vi "Thermocouple.vi"(3 "cj(mV)":dbl, 4 "factor":dbl, 5 "data":dbl) -> (0 "hot(mV)":dbl, 1 "tc(mV)":dbl, 2 "temp(degC)":dbl)   [LabVIEW 2014]
panel:
  in  "offset":dbl
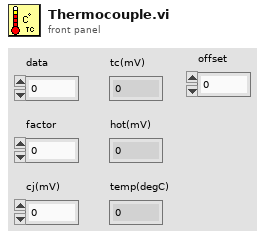
[diagram p1: front panel]
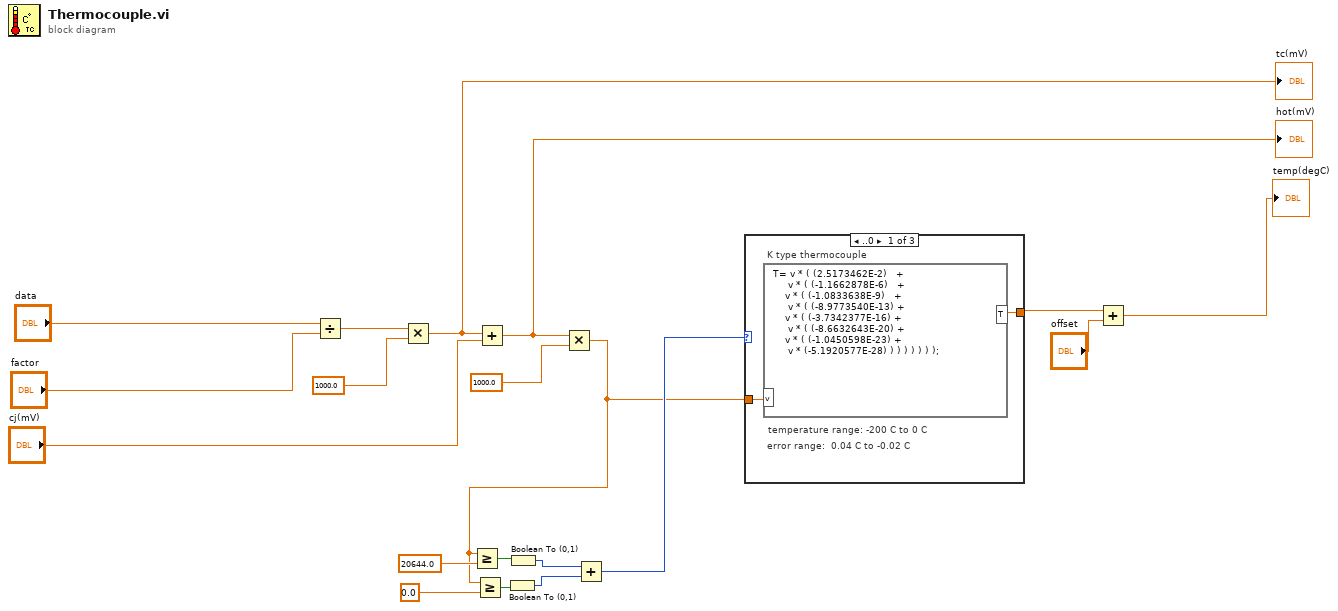
[diagram p0: block diagram]
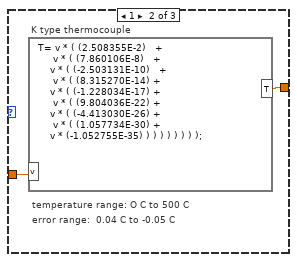
[diagram p2: hidden frame]
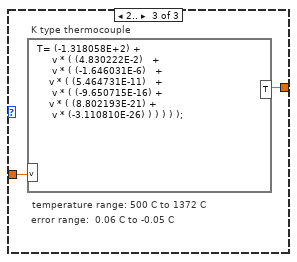
[diagram p3: hidden frame]
diagram:
  n1 = Divide(x="data", y="factor") -> (x/y=w6:dbl)
  n2 = Multiply(x=w6, y=1000.0) -> (x*y=w4:dbl)
  "tc(mV)" <- w4
  n3 = Add(x=w4, y="cj(mV)") -> (x+y=w7:dbl)
  "hot(mV)" <- w7
  n4 = Multiply(x=w7, y=1000.0) -> (x*y=w8:dbl)
  n5 = Greater Or Equal?(x=w8, y=20644.0) -> (x >= y?=w14:bool)
  n6 = Greater Or Equal?(x=w8, y=0.0) -> (x >= y?=w13:bool)
  n7 = Boolean To (0,1)(Boolean=w13) -> (0, 1=w15:i16)
  n8 = Boolean To (0,1)(Boolean=w14) -> (0, 1=w16:i16)
  n9 = Add(x=w16, y=w15) -> (x+y=w10:i16)
  n10 = case shown="..0" w10 {
    tunnel: w8 -> [w20 w22 w25]
    tunnel: [w21 w23 w24] -> w2
    frame ..0 {
      # "error range:  0.04 C to -0.02 C"
      # "temperature range: -200 C to 0 C"
      # "K type thermocouple"
      n11 = formula code="T= v * ( (2.5173462E-2)   +\n     v * ( (-1.1662878E-6)   +\n    v * ( (-1.0833638E-9)   +\n     v * ( (-8.9773540E-13) +\n    v * ( (-3.7342377E-16) +\n     v * ( (-8.6632643E-20) +\n    v * ( (-1.0450598E-23) +\n     v * (-5.1920577E-28) ) ) ) ) ) ) );"("v"=w20) -> ("T"=w21:dbl)
    }
    frame 1 {
      # "error range:  0.04 C to -0.05 C"
      # "temperature range: O C to 500 C"
      # "K type thermocouple"
      n12 = formula code="T= v * ( (2.508355E-2)   +\n     v * ( (7.860106E-8)   +\n    v * ( (-2.503131E-10)   +\n     v * ( (8.315270E-14) +\n    v * ( (-1.228034E-17) +\n     v * ( (9.804036E-22) +\n    v * ( (-4.413030E-26) +\n     v * ( (1.057734E-30) +               \n    v * (-1.052755E-35) ) ) ) ) ) ) ) );"("v"=w22) -> ("T"=w23:dbl)
    }
    frame 2.. {
      # "error range:  0.06 C to -0.05 C"
      # "temperature range: 500 C to 1372 C"
      # "K type thermocouple"
      n13 = formula code="T= (-1.318058E+2) +\n     v * ( (4.830222E-2)   +\n     v * ( (-1.646031E-6)   +\n    v * ( (5.464731E-11)   +\n     v * ( (-9.650715E-16) +\n    v * ( (8.802193E-21) +\n     v * (-3.110810E-26) ) ) ) ) );"("v"=w25) -> ("T"=w24:dbl)
    }
  }
  n14 = Add(x=w2, y="offset") -> (x+y=→"temp(degC)":dbl)
